vi "Get BIMS UDL File Path.vi"(4 "error in":errorcluster, 7 "UDL file name":path=path "BIMS_Collector.udl") -> (0 "error out":errorcluster, 2 "App.Dir":path, 3 "Full UDL file path":path)   [LabVIEW 2015]
doc: "This VI is used as a subVI in all the Database Tools example VIs. This VI looks for a file in the Examples/database directory called LabVIEW.udl and returns the path. \n\nA UDL (Universal Data Link) file specifies the connection to an OLE DB provider and a data source. The LabVIEW.udl supplied with the Database Tools examples specifies the Microsoft Jet 4.0 OLE DB Provider connected to the database file named LabVIEW.mdb."
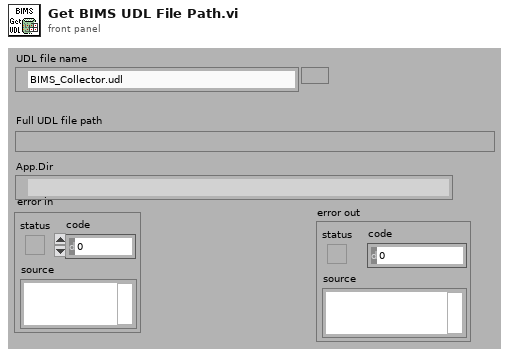
[diagram p1: front panel]
types:
  T1 = enum32{"invalid app kind", "Development System", "Run Time System", "Student Edition", "Embedded LabVIEW", "Evaluation", "Custom"}
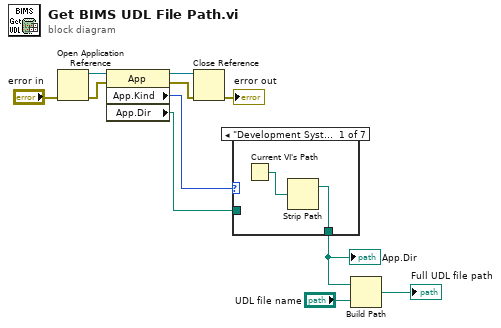
[diagram p0: block diagram]
diagram:
  n1 = Open Application Reference(8:"error in") -> (0:w7:errorcluster, 3:w8:refnum<vi>)  [unwired: 3 out]
  n2 = property class="App"(reference=w8, error in=w7) -> (reference out=w6:refnum<vi>, error out=w5:errorcluster, "App.Kind"=w4:T1, "App.Dir"=w3:path)
  n3 = Close Reference(reference=w6, error in (no error)=w5) -> (error out=→"error out":errorcluster)
  n4 = case shown="\"Development System\"" w4 {
    tunnel: [w12 w14 w15 w16 w17 w18 w19] -> w2
    tunnel: w3 -> [_ w14 w15 w16 w17 w18 w19]
    frame "Development System" {
      n5 = Current VI's Path() -> (path=w13:path)
      n6 = Strip Path(path=w13) -> (stripped path=w12:path)  [unwired: 1 out]
    }
    frame "Run Time System" {
    }
    frame "Student Edition" {
    }
    frame "Embedded LabVIEW" {
    }
    frame "Evaluation" {
    }
    frame "Custom" {
    }
    frame "invalid app kind" {
    }
  }
  "App.Dir" <- w2
  n7 = Build Path(base path=w2, name or relative path="UDL file name") -> (appended path=→"Full UDL file path":path)
